vi "feed_forward_knee.vi"(4 "fricCompV":dbl[](array[numeric]), 6 "reinitialize":bool, 7 "SetTension":dbl[](array[numeric]), 9 "limit logic in":bool[](array[boolean]), 10 "preMotorV":dbl[](array[numeric]), 11 "Constants LL":T1) -> (2 "limit logic out":bool[](array[boolean]), 3 "ff output":dbl[](array[numeric]))   [LabVIEW 2017]
uses:
  typeDef/constants_LL.ctl
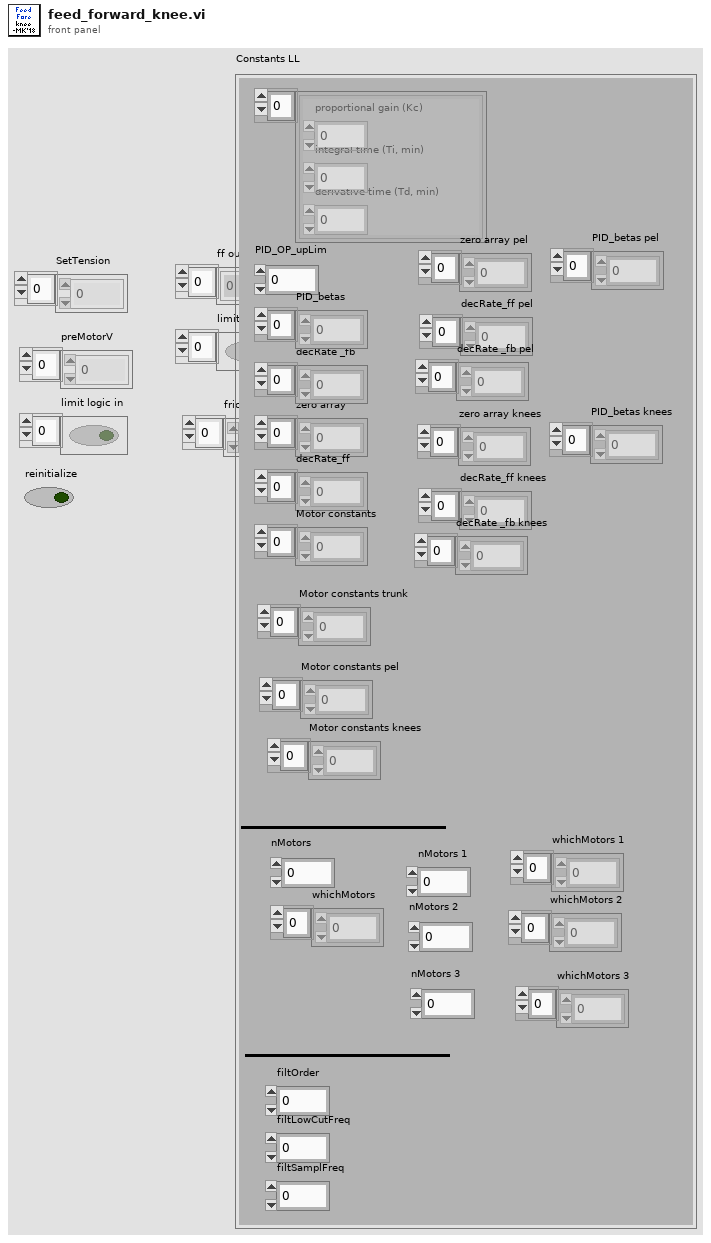
[diagram p1: front panel]
types:
  T1 = typedef "constants_LL.ctl" = cluster{"zero array":dbl[], "decRate_ff":dbl[], "Motor constants":dbl[], "PID gains":cluster{"proportional gain (Kc)":dbl, "integral time (Ti, min)":dbl, "derivative time (Td, min)":dbl}[], "decRate _fb":dbl[], "PID_OP_upLim":dbl, "nMotors":i32, "PID_betas":dbl[], "filtOrder":i32, "filtLowCutFreq":dbl, "filtSamplFreq":dbl, "whichMotors":i32[], "nMotors 1":i32, "nMotors 2":i32, "Motor constants pel":dbl[], "Motor constants trunk":dbl[], "whichMotors 1":i32[], "whichMotors 2":i32[], "zero array pel":dbl[], "decRate_ff pel":dbl[], "decRate _fb pel":dbl[], "PID_betas pel":dbl[], "whichMotors 3":i32[], "nMotors 3":i32, "Motor constants knees":dbl[], "zero array knees":dbl[], "decRate_ff knees":dbl[], "decRate _fb knees":dbl[], "PID_betas knees":dbl[]}
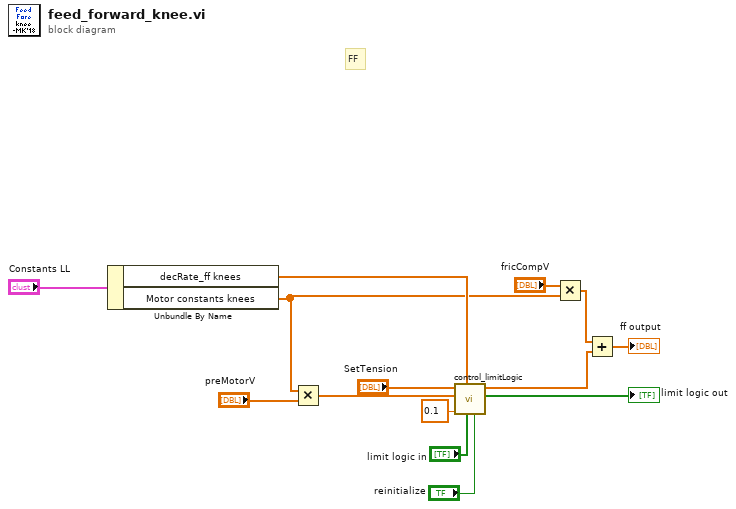
[diagram p0: block diagram]
diagram:
  # "FF"
  n1 = Unbundle By Name("Constants LL") -> ("decRate_ff knees"=w7:dbl[], "Motor constants knees"=w3:dbl[])
  n2 = Multiply(x=w3, y="preMotorV") -> (x*y=w11:dbl[])
  n3 = call "control_limitLogic.vi"("reinitialize"="reinitialize", "limit logic in"="limit logic in", "dec rate"=w7, "diff"=0.1, "Initial op"=w11, "Input"="SetTension") -> ("limit logic out"=→"limit logic out":bool[], "output"=w2:dbl[])  [unwired: 4 in]
  n4 = Multiply(x="fricCompV", y=w3) -> (x*y=w5:dbl[])
  n5 = Add(x=w5, y=w2) -> (x+y=→"ff output":dbl[])
